vi "Reset Statistics Count.vi"(8 "error in (no error)":errorcluster, 9 "Max Count (Infinite if 0)":u32, 11 "MSOX6004 in":refnum<class "MSOX6004.lvclass">) -> (0 "error out":errorcluster, 3 "MSOX6004 out":refnum<class "MSOX6004.lvclass">)   [LabVIEW 2018, in "MSOX6004.lvlib" / "MSOX6004.lvclass"]
uses:
  MSOX6004.lvclass
  MSOX6004.lvclass/MSOX6004.ctl
  <instrlib>/Keysight InfiniiVision/Keysight InfiniiVision.lvlib
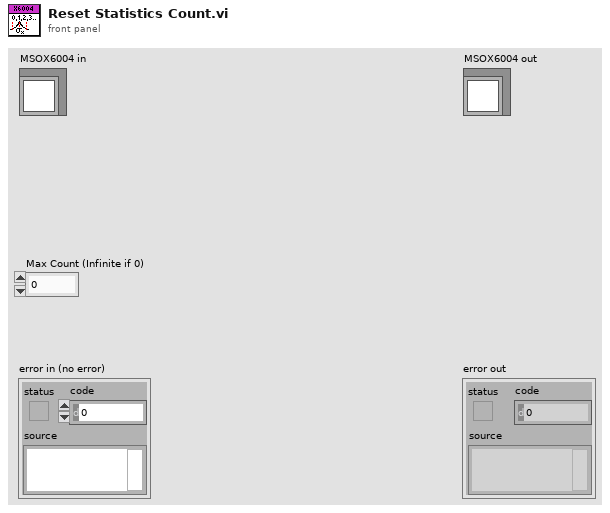
[diagram p1: front panel]
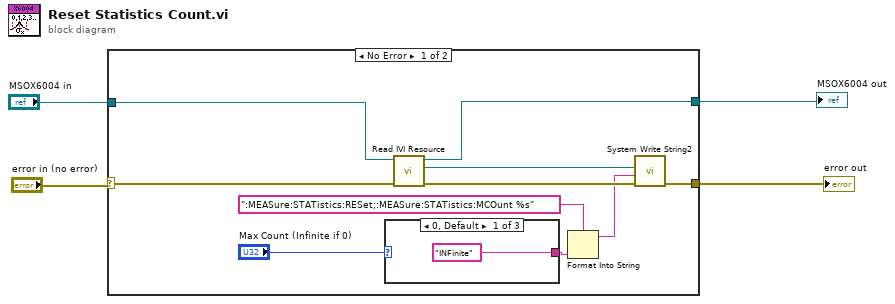
[diagram p0: block diagram]
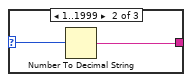
[diagram p2: hidden frame]
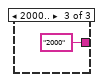
[diagram p3: hidden frame]
diagram:
  n1 = case shown="No Error" "error in (no error)" {
    selector: "error in (no error)" -> [w14 w19]
    tunnel: "MSOX6004 in" -> [w13 w20]
    tunnel: [w8 w20] -> w1
    tunnel: [w7 w19] -> w2
    frame No Error {
      n2 = case shown="0, Default" "Max Count (Infinite if 0)" {
        selector: "Max Count (Infinite if 0)" -> [_ w17 _]
        tunnel: ["INFinite" w16 "2000"] -> w5
        frame 0, Default {
        }
        frame 1..1999 {
          n3 = Number To Decimal String(number=w17) -> (decimal integer string=w16:string)  [unwired: 1 in]
        }
        frame 2000.. {
        }
      }
      n4 = call "Read IVI Resource.vi"("error in (no error)"=w14, "MSOX6004 in"=w13) -> ("error out"=w12:errorcluster, "IVI Resource"=w9:refnum<k15>, "MSOX6004 out"=w8:refnum<class "MSOX6004.lvclass">)  [unwired: 7 in]
      n5 = Format Into String(format string=":MEASure:STATistics:RESet;:MEASure:STATistics:MCOunt %s", w5) -> (resulting string=w10:string)  [unwired: 2 in, 1 out]
      n6 = call <instrlib>:"System Write String2.vi"("error in (no error)"=w12, "Data"=w10, "instrument handle"=w9) -> ("error out"=w7:errorcluster)  [unwired: 7 in, 1 out]
    }
    frame Error {
    }
  }
  "error out" <- w2
  "MSOX6004 out" <- w1
